vi "Get GUIDs for Month.vi"(8 "error in (no error)":errorcluster, 10 "Month Timestamp":timestamp=timestamp(3819510000 s since 1904-01-01) format="%<%x>T", 11 "Time Entries in":refnum<class "Time Entries.lvclass">) -> (0 "error out":errorcluster, 2 "GUIDs for Month":string[](array[string]), 3 "Time Entries out":refnum<class "Time Entries.lvclass">)   [LabVIEW 2020, in "Time Entries.lvclass"]
uses:
  Time Entries.lvclass
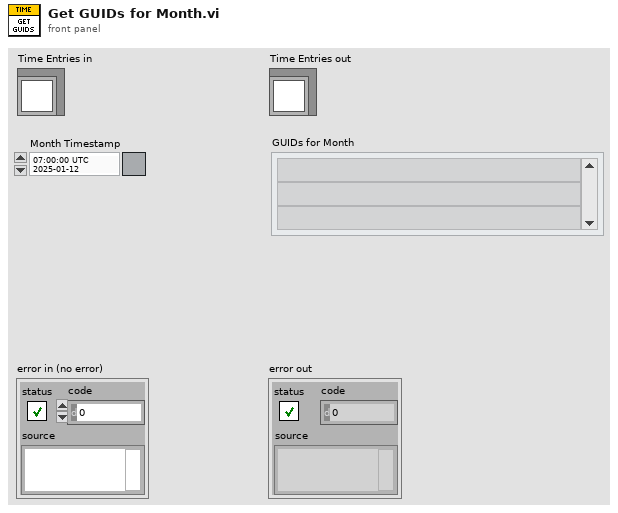
[diagram p1: front panel]
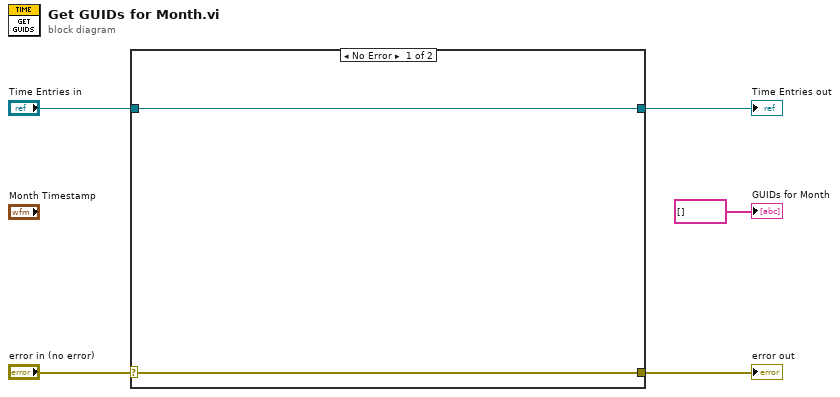
[diagram p0: block diagram]
diagram:
  n1 = case shown="No Error" "error in (no error)" {
    selector: "error in (no error)" -> [w6 w9]
    tunnel: [w6 w9] -> w4
    tunnel: [w7 w8] -> w2
    tunnel: "Time Entries in" -> [w7 w8]
    frame No Error {
    }
    frame Error {
    }
  }
  "error out" <- w4
  "Time Entries out" <- w2
  "GUIDs for Month" <- string[] [] ("GUIDs for Month")
